vi "SVFA Frequency Response (NxM) (Mag-Phase).vi"(0 "stimulus signals X [EUx]":waveform(dbl)[](array[waveform]), 1 "response signals Y [EUy]":waveform(dbl)[](array[waveform]), 2 "window":T8=1 items=["None"=0, "Hanning"=1, "Hamming"=2, "Blackman-Harris"=3, "Exact Blackman"=4, "Blackman"=5, "Flat Top"=6, "4 Term B-Harris "=7, "7 Term B-Harris"=8, "Low Sidelobe"=9, "Force - Exponential"=10, "Blackman Nuttall"=11, "Triangle"=30, "Bartlett-Hanning"=31, "Bohman"=32, "Parzen"=33, "Welch"=34, "Kaiser"=60, "Dolph-Chebyshev"=61, "Gaussian"=62], 4 "view":T11={"dB On (T)"=TRUE, "unwrap phase (F)"=FALSE, "convert to degree (T)"=TRUE}, 5 "error in (no error)":errorcluster, 6 "FRF mode":enum16{"H1", "H2", "H3"}(ring), 7 "averaging parameters":T10={"averaging mode"=enum."No averaging", "weighting mode"=enum."Exponential", "number of averages"=10, "linear mode"=enum."One shot"}, 8 "force/exp settings":T7={"force window [%]"=50.0, "exp window [%]"=10.0} {"exp window [%]" min=0.0 max=100.0 format="%.2f"; "force window [%]" min=0.0 max=100.0 format="%.2f"}, 9 "restart averaging (F)":bool) -> (11 "averaging done":bool, 12 "coherence":T9(array[cluster]) {"coherence" format="%.2f"; "df" format="%.2f"; "f0" format="%.2f"}, 13 "averages completed":dbl, 14 "magnitude [dB EUy/EUx]":T12(array[cluster]) {"magnitude" format="%.2p"; "df" format="%.2p"; "f0" format="%.2p"}, 15 "magnitude unit labels":string[][](array[string]), 16 "phase [degrees]":cluster{"f0":dbl, "df":dbl, "phase":dbl[]}[][](array[cluster]) {"phase" format="%.2f"; "df" format="%.2f"; "f0" format="%.2f"}, 17 "phase unit labels":string[][](array[string]), 18 "spectra info":T1[][](array[typedef]) {"x-axis units" items=["Time (s)"=0, "Frequency-CB (Hz)"=1, "Frequency-CPB (Hz)"=1248, "Frequency-Arbitrary (Hz)"=2357, "Quefrency (s)"=2, "Revolutions (rev)"=3, "Order"=4, "Speed (RPM)"=11, "Speed (rad/s)"=21, "Index"=65535]; "weighting filter" items=["Linear", "A-weighting", "B-weighting", "C-weighting", "ITU-R 468-4", "Dolby", "CCITT", "C-message", "Wb", "Wc", "Wd", "We", "Wf", "Wh", "Wj", "Wk", "Wm", "AES17 20 kHz lowpass", "AES17 40 kHz lowpass", "AES17 20 kHz highpass", "AES17 40 kHz highpass"]; "dB reference [EU]" format="%.2f"; "engineering units" items=["custom..."=0, "V"=1, "A"=21, "C"=30, "pC"=31, "s"=32, "-"=29, "Pa"=2, "N"=20, "g"=3, "m/s^2"=4, "m/s"=5, "m"=6, "mm/s"=12, "mm"=13, "micron/s"=14, "micron"=15, "in/s^2"=7, "in/s"=8, "in"=9, "mil/s"=10, "mil"=11, "rad/s^2"=16, "rad/s"=17, "rad"=18, "deg/s^2"=26, "deg/s"=27, "deg"=28, "RPM"=22, "cycle/s^2"=23, "Hz"=24, "cycle"=25, "strain"=19]; "spectral info"."window" items=["None "=0, "Hanning"=1, "Hamming"=2, "Blackman-Harris"=3, "Exact Blackman"=4, "Blackman"=5, "Flat Top"=6, "4 Term B-Harris "=7, "7 Term B-Harris"=8, "Low Sidelobe"=9, "Force - Exponential"=10, "Gaussian"=62]}, 19 "error out":errorcluster)   [LabVIEW 2017]
doc: "Computes the magnitude, phase, and coherence of the frequency response of the device under test [DUT]. This VI computes the ratio of the output to the input of the DUT. Wire data to the <B>stimulus signal X [Eux]</B> and <B>response signal Y [Euy]</B> inputs to determine the polymorphic instance to use or manually select the instance."
uses:
  <vilib>/addons/_NISVFA/_Shared subVIs/Controls/svc_Window [Dual FFT].ctl
  <vilib>/addons/_NISVFA/_Shared subVIs/Controls/svc_Spectrum Info.ctl
  <vilib>/addons/_NISVFA/_Shared subVIs/Controls/svc_X-Axis Units.ctl
  <vilib>/addons/_NISVFA/_Shared subVIs/Controls/svc_Spectrum Type.ctl
  <vilib>/addons/_NISVFA/_Shared subVIs/Controls/svc_Engineering Units Text Ring.ctl
  <vilib>/addons/_NISVFA/_Shared subVIs/Controls/svc_Weighting Filter Text Ring.ctl
  <vilib>/addons/_NISVFA/_Shared subVIs/Controls/svc_Complimentary Spectrum Units.ctl
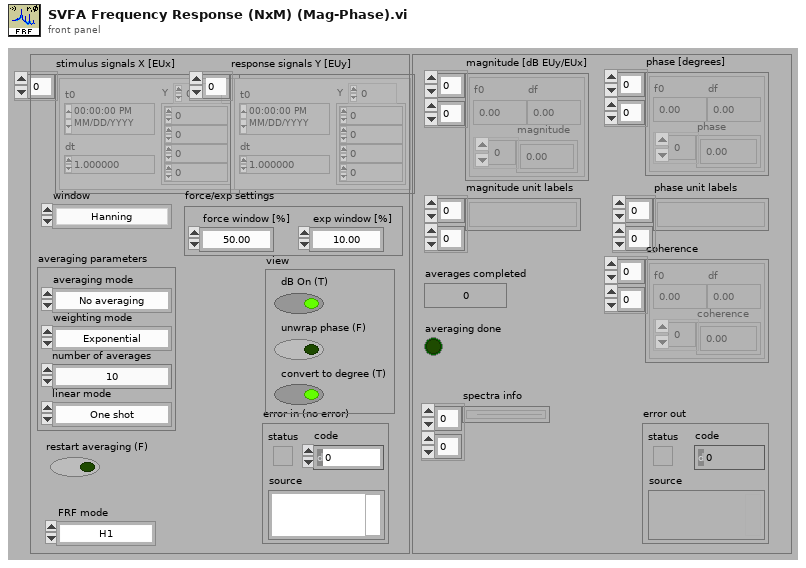
[diagram p1: front panel]
types:
  T1 = typedef "svc_Spectrum Info.ctl" = cluster{"channel name":string, "description":string, "x-axis units":T2, "spectral info":cluster{"spectrum type":T3, "linear/dB":enum16{"linear", "dB"}, "window":u16, "window size":i32, "FFT size":i32}, "engineering units":T4, "custom label":string, "dB reference [EU]":dbl, "peak units":enum16{"rms", "peak", "peak-peak"}, "weighting filter":T5, "spectral density?":bool, "unit label":string, "spectrum skewed?":bool, "complimentary spectrum units":T6}
  T2 = typedef "svc_X-Axis Units.ctl" = u16
  T3 = typedef "svc_Spectrum Type.ctl" = enum16{"FFT Spectrum [complex]", "Amplitude [Magnitude]", "Power [Magnitude^2]", "Cross Spectrum [complex]", "Frequency Response [Complex]"}
  T4 = typedef "svc_Engineering Units Text Ring.ctl" = u16
  T5 = typedef "svc_Weighting Filter Text Ring.ctl" = u16
  T6 = typedef "svc_Complimentary Spectrum Units.ctl" = enum16{"none", "radians", "degrees", "cycles", "imaginary"}
  T7 = cluster{"force window [%]":dbl, "exp window [%]":dbl}
  T8 = typedef "svc_Window [Dual FFT].ctl" = u32
  T9 = cluster{"f0":dbl, "df":dbl, "coherence":dbl[]}[][]
  T10 = cluster{"averaging mode":enum16{"No averaging", "Vector averaging", "RMS averaging", "Peak hold"}, "weighting mode":enum16{"Linear", "Exponential"}, "number of averages":u32, "linear mode":enum16{"One shot", "Auto restart"}}
  T11 = cluster{"dB On (T)":bool, "unwrap phase (F)":bool, "convert to degree (T)":bool}
  T12 = cluster{"f0":dbl, "df":dbl, "magnitude":dbl[]}[][]
  T13 = enum16{"Cross spectrum", "Frequency response", "Coherent output power"}
  T14 = enum16{"Restart processing", "Continue processing", "Skip processing"}
  T15 = cluster{"f0":dbl, "df":dbl, "complex spectrum":cdb[]}[][]
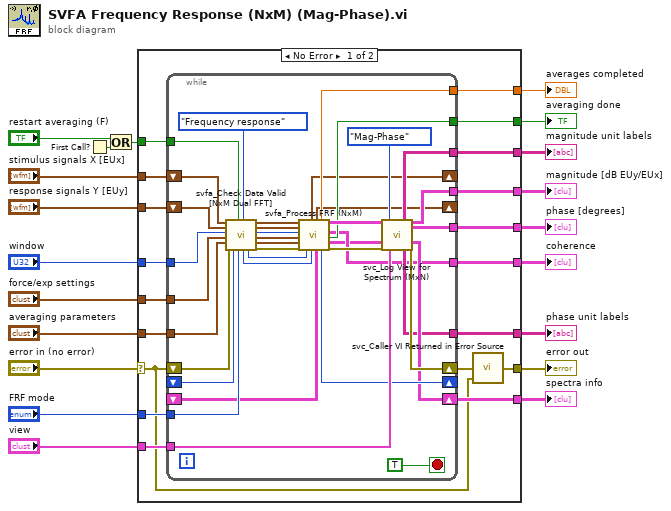
[diagram p0: block diagram]
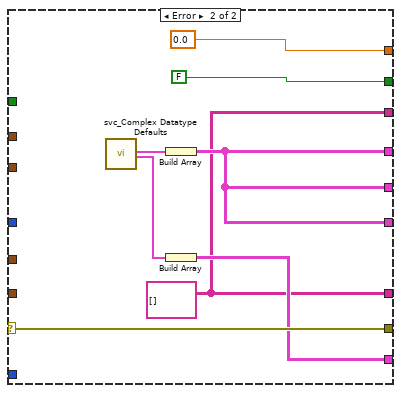
[diagram p2: hidden frame]
diagram:
  n1 = First Call?() -> (First Call?: T/F=w4:bool)
  n2 = Or(x="restart averaging (F)", y=w4) -> (x .or. y?=w3:bool)
  n3 = case shown="No Error" "error in (no error)" {
    selector: "error in (no error)" -> [w21 w84]
    tunnel: "averaging parameters" -> [w29 _]
    tunnel: "window" -> [w30 _]
    tunnel: "force/exp settings" -> [w28 _]
    tunnel: "stimulus signals X [EUx]" -> [w39 _]
    tunnel: "response signals Y [EUy]" -> [w38 _]
    tunnel: [w35 w80] -> w14
    tunnel: [w34 w80] -> w13
    tunnel: [w32 w80] -> w12
    tunnel: [w23 w84] -> w11
    tunnel: [w37 FALSE ("averaging done")] -> w10
    tunnel: [w36 0.0 ("averages completed")] -> w9
    tunnel: w3 -> [w24 _]
    tunnel: "view" -> [w31 _]
    tunnel: "FRF mode" -> [w27 _]
    tunnel: [w22 w78] -> w1
    tunnel: [w26 w77] -> w6
    tunnel: [w25 w77] -> w5
    frame No Error {
      n4 = while {
        tunnel: w24 -> [w50]
        tunnel: [w52] -> w25
        tunnel: [w53] -> w26
        shift-left: _ -> [w51]
        shift-right: [w56] -> _
        tunnel: w27 -> [w48]
        tunnel: w28 -> [w65]
        tunnel: w29 -> [w63]
        tunnel: w30 -> [w66]
        tunnel: w31 -> [w67]
        tunnel: [w46] -> w32
        tunnel: [w69] -> w34
        tunnel: [w70] -> w35
        tunnel: [w72] -> w36
        tunnel: [w55] -> w37
        shift-right: [w68] -> w33
        shift-left: w21 -> [w76]
        shift-right: [w43] -> _
        shift-left: w39 -> [w75]
        shift-right: [w44] -> _
        shift-left: w38 -> [w74]
        shift-right: [w54] -> w22
        shift-left: _ -> [w42]
        stop <- TRUE stop-if-true
        n5 = call <vilib>:"svfa_Check Data Valid [NxM Dual FFT].vi"("stimulus signals X [EUx]"=w75, "response signals Y [EUy]"=w74, "window"=w66, "force/exp settings"=w65, "averaging parameters"=w63, "error in (no error)"=w76, "processing control in"=w51, "restart averaging (F)"=w50, "FRF mode"=w48, "measurement"=T13."Frequency response") -> ("dup FRF mode"=w47:enum16{"H1", "H2", "H3"}, "processing control out"=w40:T14, "dup stimulus signals X [EUx]"=w62:waveform(dbl)[], "response signals Y [EUy]"=w61:waveform(dbl)[], "window"=w60:T8, "dup force/exp settings"=w59:T7, "dup averaging parameters"=w58:T10, "error out"=w57:errorcluster)  [unwired: 2 in]
        n6 = call <vilib>:"svfa_Process FRF (NxM).vi"("stimulus signals X [EUx]"=w62, "response signals Y [EUy]"=w61, "window"=w60, "force/exp settings"=w59, "averaging parameters"=w58, "error in (no error)"=w57, "processing control"=w40, "FRF mode"=w47, "spectra info in"=w42) -> ("stimulus signals X [EUx] 2"=w43:waveform(dbl)[], "response signals Y [EUy] 2"=w44:waveform(dbl)[], "averages completed"=w72:dbl, "processing control"=w56:T14, "complex responses [EUy/EUx]"=w71:T15, "coherence"=w46:T9, "averaging done"=w55:bool, "spectra info out"=w45:T1[][], "error out"=w73:errorcluster)  [unwired: 2 in]
        n7 = call <vilib>:"svc_Log View for Spectrum (MxN).vi"("complex responses [EUy/EUx]"=w71, "spectra info in"=w45, "error in (no error)"=w73, 6:"view"=enum16{"Mag-Phase", "Real-Imaginary"}."Mag-Phase" ("View"), 7:"view"=w67) -> ("unit labels (mag or real)"=w53:string[][], "unit labels (phase or imag)"=w52:string[][], "magnitudes [dB EUy/EUx]"=w70:T12, "phases [degree]"=w69:cluster{"f0":dbl, "df":dbl, "phase":dbl[]}[][], "spectra info out"=w54:T1[][], "error out"=w68:errorcluster)  [unwired: 9 in]
      }
      n8 = call <vilib>:"svc_Caller VI Returned in Error Source.vi"("warning input to caller"=w21, "error in (no error)"=w33) -> ("error out"=w23:errorcluster)  [unwired: 3 in]
    }
    frame Error {
      w77 = string[][] []
      n9 = call <vilib>:"svc_Complex Datatype Defaults.vi"() -> ("empty array of spectra"=w81:cluster{"f0":dbl, "df":dbl, "magnitude":dbl[]}[], "empty array of spectrum info"=w79:T1[])  [unwired: 11 in, 7 out]
      n10 = Build Array(w81) -> (w80:T12)
      n11 = Build Array(w79) -> (w78:T1[][])
    }
  }
  "error out" <- w11
  "magnitude [dB EUy/EUx]" <- w14
  "phase [degrees]" <- w13
  "averaging done" <- w10
  "averages completed" <- w9
  "coherence" <- w12
  "spectra info" <- w1
  "phase unit labels" <- w5
  "magnitude unit labels" <- w6
